vi "Configure Measurement (Edge Time).vi"(5 "Upper Reference Value (4.0 V)":dbl=4.0 format="%#_4g", 7 "Lower Reference Value (-4.0 V)":dbl=-4.0 format="%#_4g", 8 "error in (no error)":errorcluster, 9 "Edge Time Type (0:Rise)":i32(ring) items=["Rise", "Fall"], 10 "Channel (1:Channel 1)":i32(ring)=1 items=["Channel 1"=1, "Channel 2"=2], 11 "VISA resource name":refnum<visa-resource-name>) -> (0 "error out":errorcluster, 3 "VISA resource name out":refnum<visa-resource-name>)   [LabVIEW 2015, in "Template - Counter.lvlib"]
doc: "Configures the settings required for Edge Time measurements."
uses:
  <instrlib>/_Template - Counter/Template - Counter.lvlib
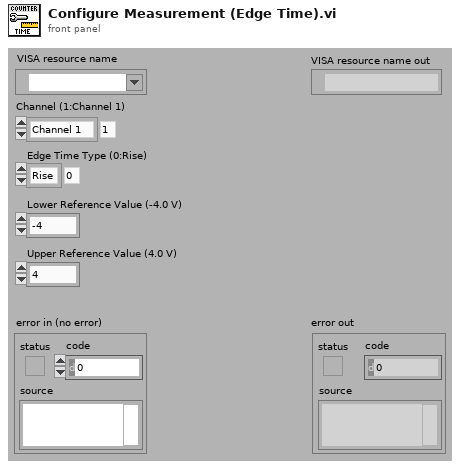
[diagram p1: front panel]
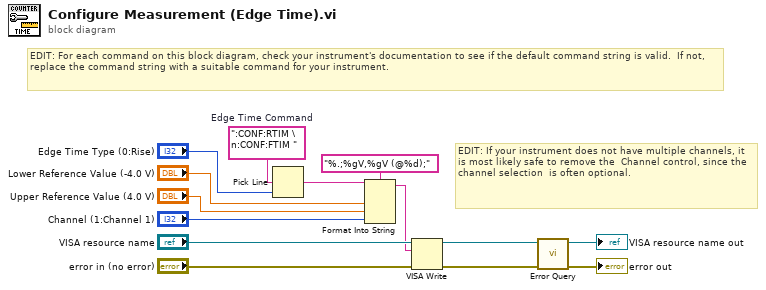
[diagram p0: block diagram]
diagram:
  w8 = ":CONF:RTIM \n:CONF:FTIM "  # Edge Time Command
  # "EDIT: If your instrument does not have multiple channels, it is most likely safe to remove the  Channel control, since the channel selection  is often optional."
  # "EDIT: For each command on this block diagram, check your instrument's documentation to see if the default command string is valid.  If not, replace the command string with a suitable command for your instrument."
  n1 = Pick Line(multi-line string=w8, line index="Edge Time Type (0:Rise)") -> (output string=w3:string)  [unwired: 1 in]
  n2 = Format Into String(format string="%.;%gV,%gV (@%d);", initial string=w3, "Lower Reference Value (-4.0 V)", "Upper Reference Value (4.0 V)", "Channel (1:Channel 1)") -> (resulting string=w2:string)  [unwired: 1 in, 1 out]
  n3 = VISA Write(VISA resource name="VISA resource name", write buffer=w2, error in (no error)="error in (no error)") -> (VISA resource name out=w12:refnum<visa-resource-name>, error out=w10:errorcluster)  [unwired: 1 out]
  n4 = call <instrlib>:"Error Query.vi"("error in (no error)"=w10, "VISA resource name"=w12) -> ("error out"=→"error out":errorcluster, "VISA resource name out"=→"VISA resource name out":refnum<visa-resource-name>)  [unwired: 6 in, 2 out]
